vi "crio_RT_Antagonist_Depre.vi"() -> ()   [LabVIEW 2019]
uses:
  <vilib>/rvi/interface/nirviReadWriteControl/nirviReadWriteControl.xnode
  <vilib>/rvi/interface/Simulation/niFpgaSimulationCallBeginRW.vi
  <vilib>/rvi/errors/niLvFpgaAdjustHostInterfaceError.vi
  <vilib>/ptbypt/NI_PtbyPt.lvlib
  <vilib>/rvi/interface/nirviCloseFPGA/nirviCloseFPGA.xnode
  NiFpgaLv.dll
  <vilib>/Utility/error.llb/Error Cluster From Error Code.vi
  <vilib>/rvi/interface/nirviMethod/nirviMethod.xnode
  <vilib>/FPGAPlugInAG/Dynamic/niLvFpga_ReadFifo_Dynamic.vi
  <vilib>/rvi/errors/niLvFpgaMergeErrorWithErrorCode.vi
  <vilib>/rvi/interface/nirviOpenFPGA/nirviOpenFPGA.xnode
  FPGA Bitfiles/gpass2_FPGATarget2_crioFPGAAntagoni_cDOKBUczdNQ.lvbitx
  crio_FPGA_Antagonist.vi
  <vilib>/FPGAPlugInAG/cRIO-9074/niLvFpga_Open_cRIO-9074.vi
  <vilib>/rvi/interface/common/dynamic/niFpgaDynamicAddResources.vi
  <vilib>/FPGAPlugInAG/Dynamic/niLvFpga_Close_Dynamic.vi
panel:
  out "Commanded LAC Position":sgl
  in  "LAC position (fully 0: retract, 1: extend)":sgl(slide) scale=0.0..1.0
  in  "stop":bool
  out "FIFO Data":i32(graph)
  out "Computed Bias":dbl(graph)
  out "Offsetted Data":dbl(graph)
  out "HX711 Raw Data":i32(graph)
  in  "FIFO Element Threshold":u32
  out "HX711 FIFO Data":i32[](array[numeric])
  out "HX711 Raw Data":i32
  in  "Gain/ChannelSelect":T1(ring)=enum."Channel A/Gain 64"
  out "Computed Bias":dbl format="%0.2f"
  in  "Number of Samples for Offset Computation":i32=100
  in  "Offset Bias":bool
  out "Offsetted Data":dbl
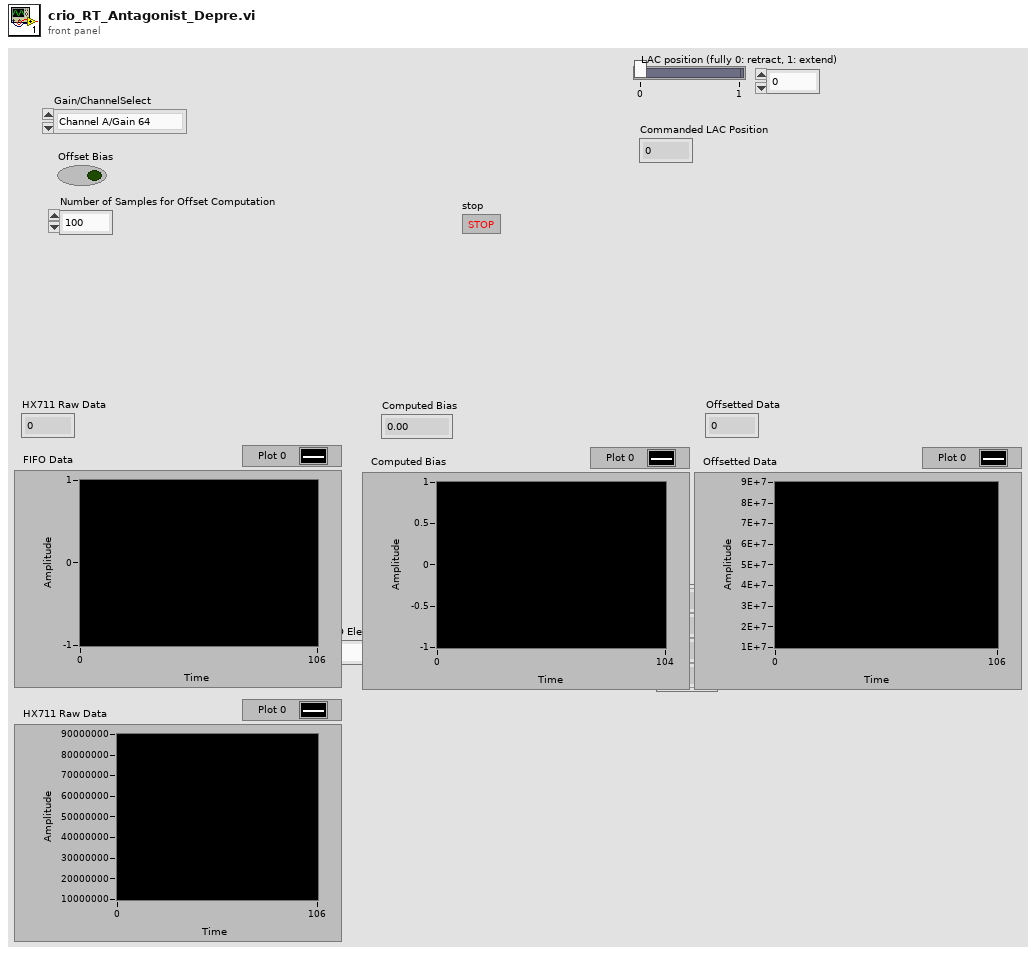
[diagram p1: front panel]
types:
  T1 = enum16{"Channel A/Gain 128", "Channel A/Gain 64", "Channel B/Gain 32"}
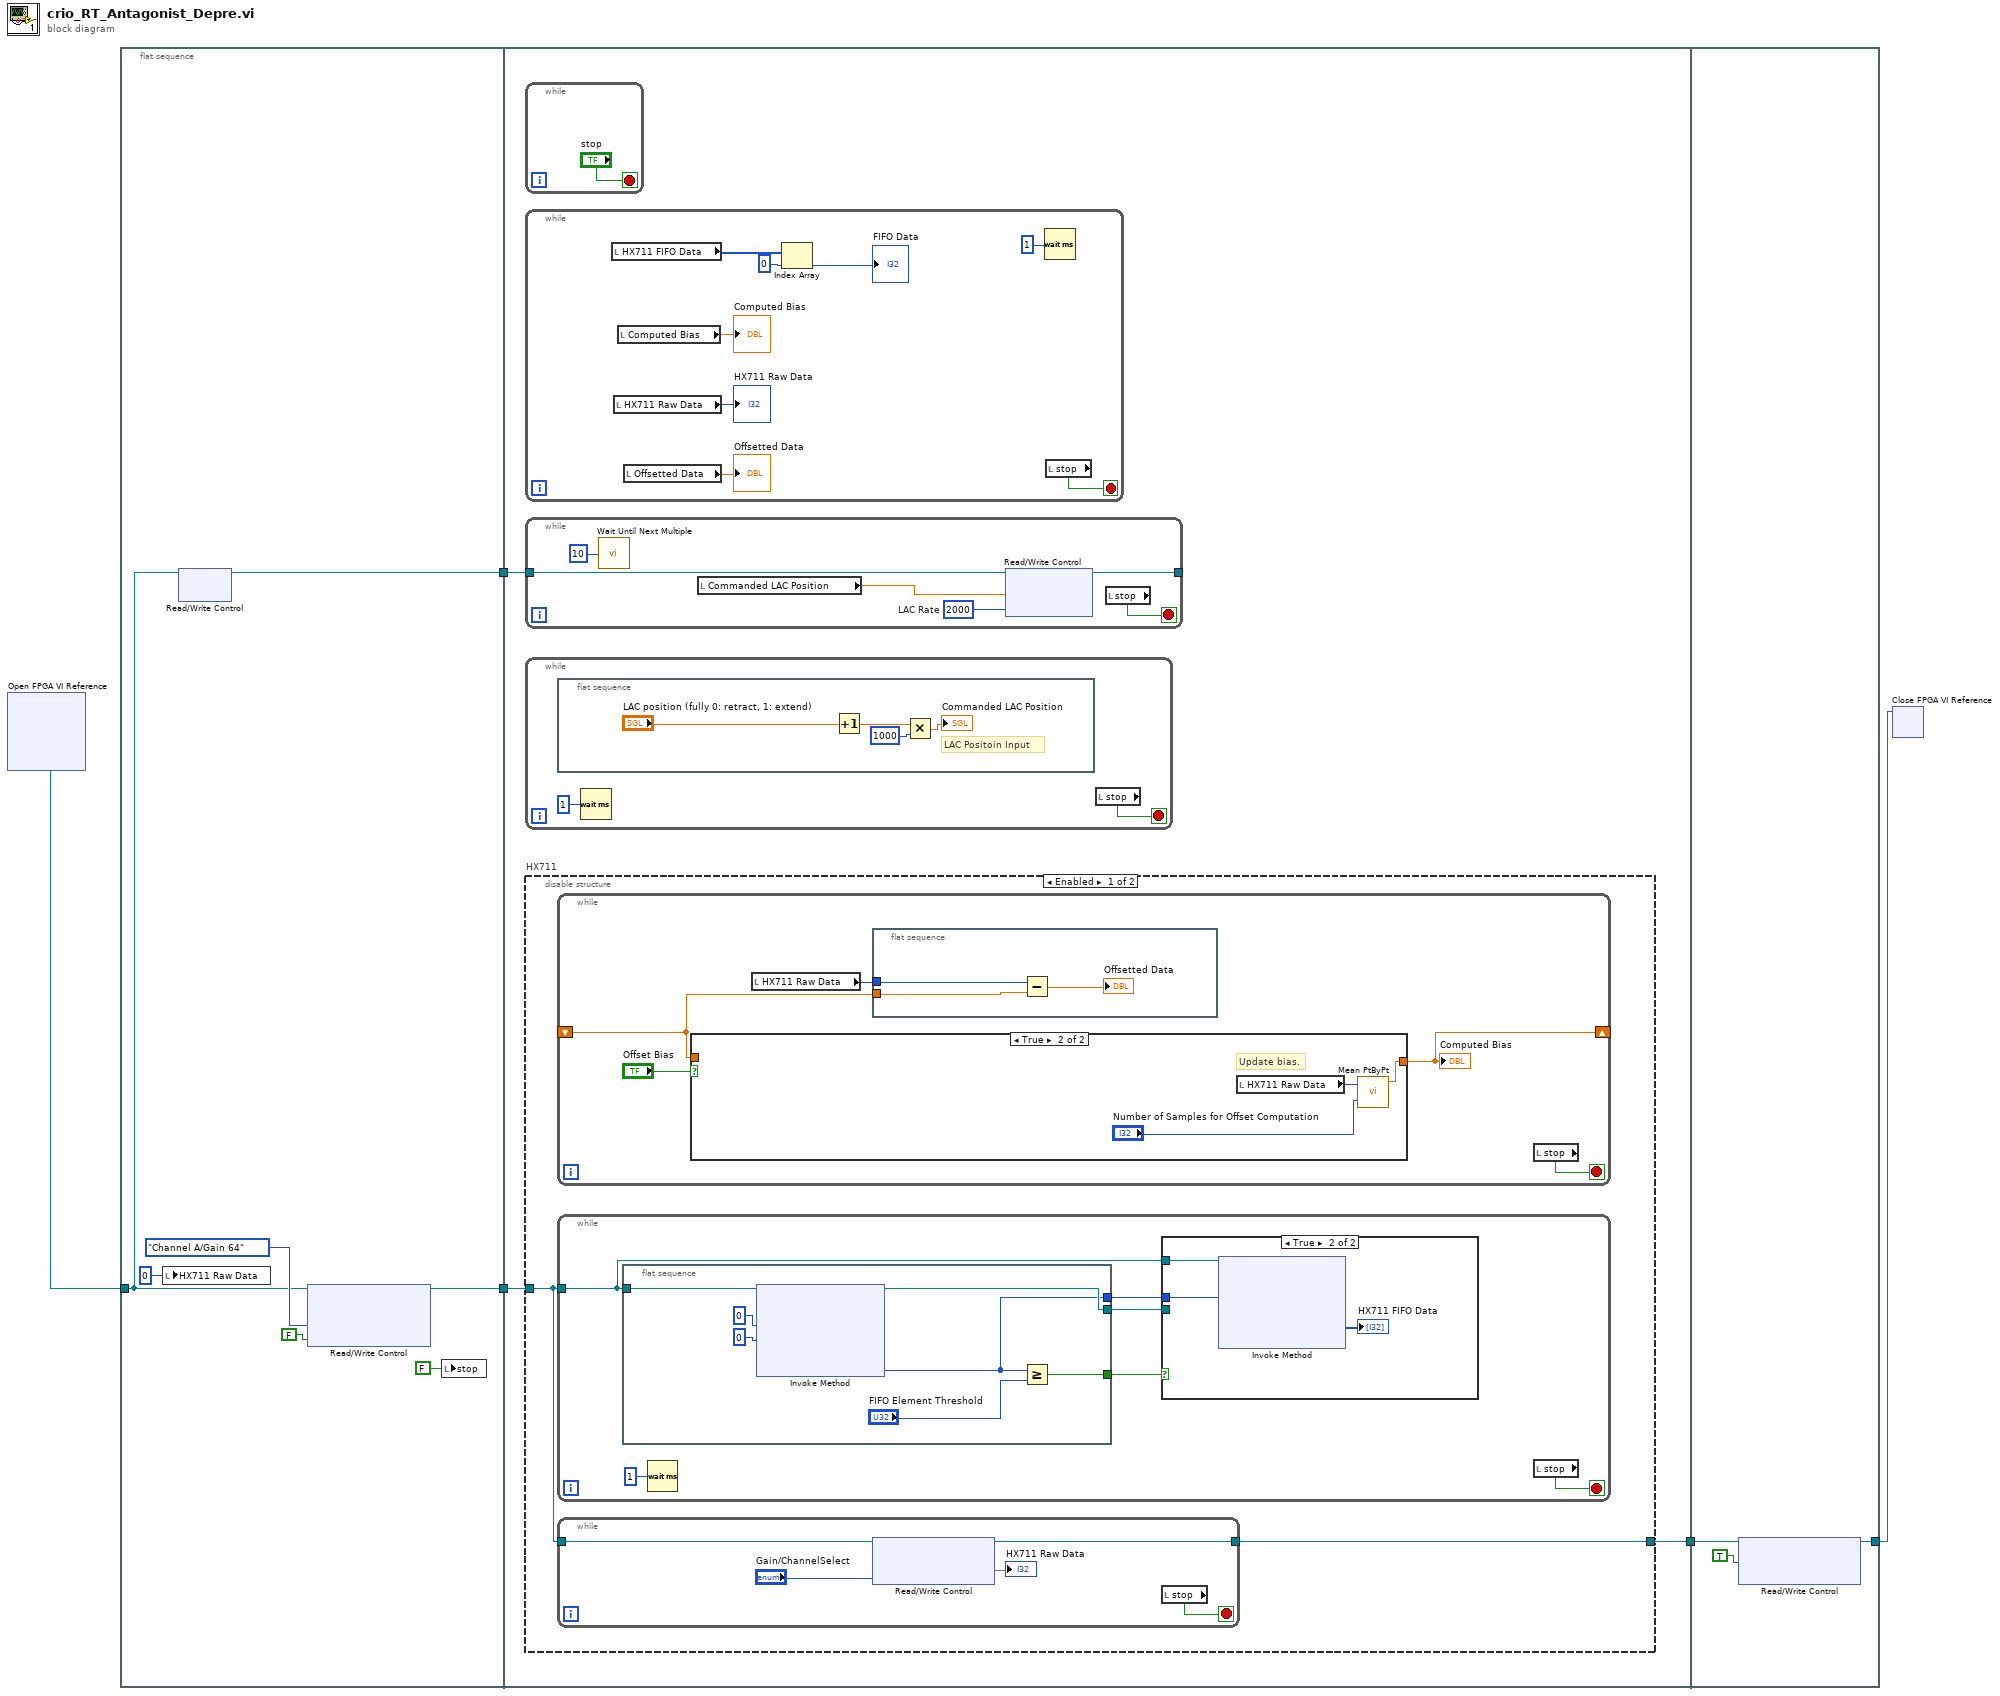
[diagram p0: block diagram]
diagram:
  n1 = xnode "Open FPGA VI Reference"() -> ("FPGA VI Reference Out"=w2:refnum<k20>)  [unwired: 2 in, 1 out]
  n2 = flat-sequence {
    tunnel: [w10] -> w5
    tunnel: w2 -> [w7]
    tunnel: [w6] -> w1
    tunnel: w5 -> [w14]
    tunnel: [w15] -> w4
    tunnel: w1 -> [w13]
    tunnel: w4 -> [w73]
    tunnel: [w72] -> w3
    frame #0 {
      n3 = local write "HX711 Raw Data"(0 ("Data")) -> ()
      n4 = xnode "Read/Write Control"("FPGA VI Reference In"=w7) -> ("FPGA VI Reference Out"=w6:refnum<k20>)  [unwired: 1 in, 2 out]
      n5 = xnode "Read/Write Control"("FPGA VI Reference In"=w7, "Gain/ChannelSelect"=T1."Channel A/Gain 64", "stop"=FALSE) -> ("FPGA VI Reference Out"=w10:refnum<k20>)  [unwired: 1 in, 2 out]
      n6 = local write "stop"(FALSE ("stop")) -> ()
    }
    frame #1 {
      n7 = while {
        stop <- "stop" stop-if-true
      }
      n8 = while {
        stop <- w23 stop-if-true
        n9 = local read "HX711 FIFO Data"() -> (w19:i32[])
        n10 = local read "HX711 Raw Data"() -> (→"HX711 Raw Data":i32)
        n11 = local read "Computed Bias"() -> (→"Computed Bias":dbl)
        n12 = local read "Offsetted Data"() -> (→"Offsetted Data":dbl)
        n13 = Index Array(array=w19, index=0) -> (element=→"FIFO Data":i32)
        n14 = Wait (ms)(milliseconds to wait=u32 1) -> ()  [unwired: 1 out]
        n15 = local read "stop"() -> (w23:bool)
      }
      n16 = while {
        tunnel: w13 -> [w35]
        tunnel: [w34] -> _
        stop <- w31 stop-if-true
        w33 = u32 2000  # LAC Rate
        n17 = call "Wait Until Next Multiple"("Count(mSec)"=u32 10) -> ()  [unwired: 1 out]
        n18 = local read "Commanded LAC Position"() -> (w30:sgl)
        n19 = xnode "Read/Write Control"("FPGA VI Reference In"=w35, "LAC Position"=w30, "Count(uSec)"=w33) -> ("FPGA VI Reference Out"=w34:refnum<k20>)  [unwired: 1 in, 1 out]
        n20 = local read "stop"() -> (w31:bool)
      }
      n21 = while {
        stop <- w25 stop-if-true
        n22 = flat-sequence {
          frame #0 {
            # "LAC Positoin Input"
            n23 = Increment(x="LAC position (fully 0: retract, 1: extend)") -> (x+1=w28:sgl)
            n24 = Multiply(x=w28, y=i16 1000) -> (x*y=→"Commanded LAC Position":sgl)
          }
        }
        n25 = Wait (ms)(milliseconds to wait=u32 1) -> ()  [unwired: 1 out]
        n26 = local read "stop"() -> (w25:bool)
      }
      n27 = disable-structure "HX711" shown="Enabled" {
        disable-tunnel: [w37 _] -> w15
        disable-tunnel: w14 -> [w36 _]
        frame Enabled {
          n28 = while {
            shift-right: [w56] -> _
            shift-left: _ -> [w54]
            stop <- w58 stop-if-true
            n29 = case shown="True" "Offset Bias" {
              tunnel: [w62 w64] -> w56
              tunnel: w54 -> [w62 _]
              frame False {
                # "Stick with latest bias."
              }
              frame True {
                # "Update bias."
                n30 = local read "HX711 Raw Data"() -> (w65:i32)
                n31 = call <vilib>:"Mean PtByPt.vi"("x"=w65, "sample length"="Number of Samples for Offset Computation") -> ("mean"=w64:dbl)  [unwired: 2 in, 1 out]
              }
            }
            "Computed Bias" <- w56
            n32 = local read "HX711 Raw Data"() -> (w55:i32)
            n33 = flat-sequence {
              tunnel: w55 -> [w61]
              tunnel: w54 -> [w60]
              frame #0 {
                n34 = Subtract(x=w61, y=w60) -> (x-y=→"Offsetted Data":dbl)
              }
            }
            n35 = local read "stop"() -> (w58:bool)
          }
          n36 = while {
            tunnel: w36 -> [w43]
            stop <- w41 stop-if-true
            n37 = flat-sequence {
              tunnel: w43 -> [w53]
              tunnel: [w51] -> w42
              tunnel: [w50] -> w40
              tunnel: [w49] -> w39
              frame #0 {
                n38 = xnode "Invoke Method"("FPGA VI Reference In"=w53, "Number of Elements"=0 ("Timeout (ms)"), "Timeout (ms)"=u32 0 ("Number of Elements")) -> ("FPGA VI Reference Out"=w51:refnum<k20>, "Elements Remaining"=w49:u32)  [unwired: 1 in, 2 out]
                n39 = Greater Or Equal?(x=w49, y="FIFO Element Threshold") -> (x >= y?=w50:bool)
              }
            }
            n40 = Wait (ms)(milliseconds to wait=u32 1) -> ()  [unwired: 1 out]
            n41 = case shown="True" w40 {
              tunnel: w43 -> [_ w46]
              tunnel: w42 -> [_ _]
              tunnel: w39 -> [_ w45]
              frame False {
              }
              frame True {
                n42 = xnode "Invoke Method"("FPGA VI Reference In"=w46, "Number of Elements"=w45) -> ("Data"=→"HX711 FIFO Data":i32[])  [unwired: 2 in, 3 out]
              }
            }
            n43 = local read "stop"() -> (w41:bool)
          }
          n44 = while {
            tunnel: w36 -> [w70]
            tunnel: [w67] -> w37
            stop <- w66 stop-if-true
            n45 = xnode "Read/Write Control"("FPGA VI Reference In"=w70, "Gain/ChannelSelect"="Gain/ChannelSelect") -> ("FPGA VI Reference Out"=w67:refnum<k20>, "Data"=→"HX711 Raw Data")  [unwired: 1 in, 1 out]
            n46 = local read "stop"() -> (w66:bool)
          }
        }
        frame Disabled {
        }
      }
    }
    frame #2 {
      n47 = xnode "Read/Write Control"("FPGA VI Reference In"=w73, "stop"=TRUE) -> ("FPGA VI Reference Out"=w72:refnum<k20>)  [unwired: 2 in, 1 out]
    }
  }
  n48 = xnode "Close FPGA VI Reference"("FPGA VI Reference In"=w3) -> ()  [unwired: 1 in, 1 out]
